vi "valve_command.vi"(8 "Error IN":errorcluster, 9 "Command option":string, 10 "COMMANDS":T1(ring), 11 "VALVE PORT IN":refnum<visa-resource-name>="COM1") -> (0 "Error OUT":errorcluster, 2 "read buffer":string, 3 "VALVE PORT OUT":refnum<visa-resource-name>)   [LabVIEW 2013]
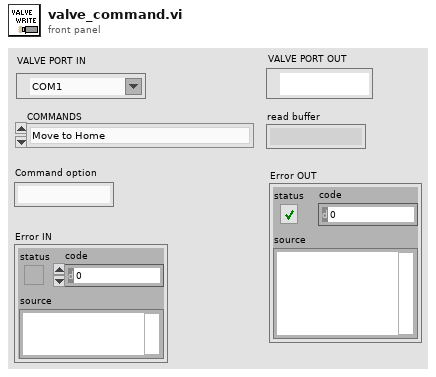
[diagram p1: front panel]
types:
  T1 = enum16{"Move to Home", "Set Positions", "Set Actuator Mode", "OTHER", "Set Direction", "CW Move", "CCW Move"}
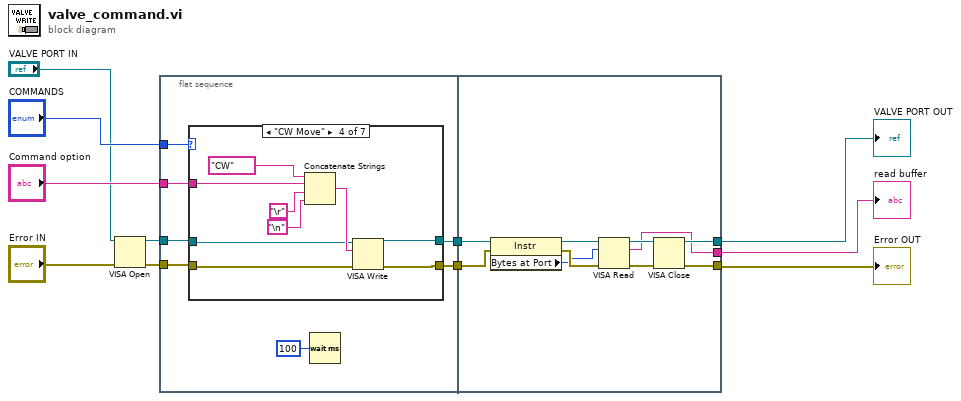
[diagram p0: block diagram]
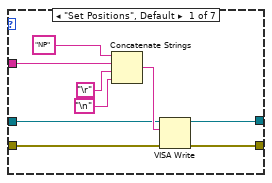
[diagram p2: hidden frame]
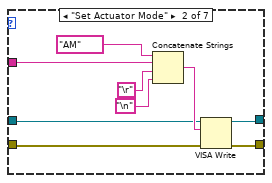
[diagram p3: hidden frame]
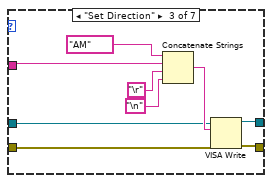
[diagram p4: hidden frame]
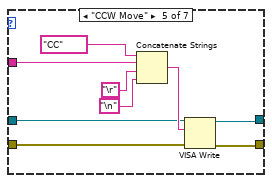
[diagram p5: hidden frame]
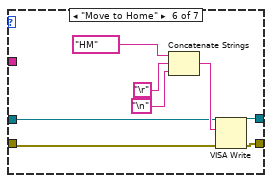
[diagram p6: hidden frame]
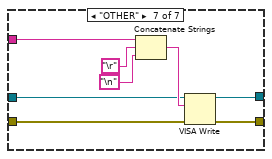
[diagram p7: hidden frame]
diagram:
  n1 = VISA Open(error in (no error)="Error IN", VISA resource name="VALVE PORT IN") -> (VISA resource name=w6:refnum<visa-resource-name>, error out=w4:errorcluster)  [unwired: 3 in]
  n2 = flat-sequence {
    tunnel: "COMMANDS" -> [w18]
    tunnel: "Command option" -> [w17]
    tunnel: w6 -> [w14]
    tunnel: w4 -> [w13]
    tunnel: [w16] -> w3
    tunnel: [w15] -> w2
    tunnel: [w81] -> w8
    tunnel: [w82] -> w9
    tunnel: w3 -> [w83]
    tunnel: w2 -> [w84]
    tunnel: [w80] -> w1
    frame #0 {
      n3 = case shown="\"CW Move\"" w18 {
        tunnel: w14 -> [w21 w29 w41 w49 w59 w69 w75]
        tunnel: w13 -> [w23 w32 w40 w48 w58 w66 w74]
        tunnel: w17 -> [w19 w28 w37 w50 w55 _ w78]
        tunnel: [w20 w30 w38 w46 w57 w68 w73] -> w15
        tunnel: [w22 w31 w39 w47 w56 w67 w72] -> w16
        frame "Set Positions", Default {
          n4 = Concatenate Strings("NP" ("write buffer 2"), w19, "\r", "\n") -> (w27:string)
          n5 = VISA Write(VISA resource name=w21, write buffer=w27, error in (no error)=w23) -> (VISA resource name out=w20:refnum<visa-resource-name>, error out=w22:errorcluster)  [unwired: 1 out]
        }
        frame "Set Actuator Mode" {
          n6 = Concatenate Strings("AM" ("write buffer 2"), w28, "\r", "\n") -> (w33:string)
          n7 = VISA Write(VISA resource name=w29, write buffer=w33, error in (no error)=w32) -> (VISA resource name out=w30:refnum<visa-resource-name>, error out=w31:errorcluster)  [unwired: 1 out]
        }
        frame "Set Direction" {
          n8 = Concatenate Strings("AM" ("write buffer 2"), w37, "\r", "\n") -> (w42:string)
          n9 = VISA Write(VISA resource name=w41, write buffer=w42, error in (no error)=w40) -> (VISA resource name out=w38:refnum<visa-resource-name>, error out=w39:errorcluster)  [unwired: 1 out]
        }
        frame "CW Move" {
          n10 = Concatenate Strings("CW" ("write buffer 2"), w50, "\r", "\n") -> (w51:string)
          n11 = VISA Write(VISA resource name=w49, write buffer=w51, error in (no error)=w48) -> (VISA resource name out=w46:refnum<visa-resource-name>, error out=w47:errorcluster)  [unwired: 1 out]
        }
        frame "CCW Move" {
          n12 = Concatenate Strings("CC" ("write buffer 2"), w55, "\r", "\n") -> (w60:string)
          n13 = VISA Write(VISA resource name=w59, write buffer=w60, error in (no error)=w58) -> (VISA resource name out=w57:refnum<visa-resource-name>, error out=w56:errorcluster)  [unwired: 1 out]
        }
        frame "Move to Home" {
          n14 = Concatenate Strings("HM" ("write buffer 2"), "\r", "\n") -> (w71:string)
          n15 = VISA Write(VISA resource name=w69, write buffer=w71, error in (no error)=w66) -> (VISA resource name out=w68:refnum<visa-resource-name>, error out=w67:errorcluster)  [unwired: 1 out]
        }
        frame "OTHER" {
          n16 = Concatenate Strings(w78, "\r", "\n") -> (w79:string)
          n17 = VISA Write(VISA resource name=w75, write buffer=w79, error in (no error)=w74) -> (VISA resource name out=w73:refnum<visa-resource-name>, error out=w72:errorcluster)  [unwired: 1 out]
        }
      }
      n18 = Wait (ms)(milliseconds to wait=u32 100) -> ()  [unwired: 1 out]
    }
    frame #1 {
      n19 = property class="Instr"(reference=w84, error in=w83) -> (reference out=w86:refnum<visa-resource-name>, error out=w87:errorcluster, "Bytes at Port"=w85:u32)
      n20 = VISA Read(VISA resource name=w86, byte count=w85, error in (no error)=w87) -> (VISA resource name out=w81:refnum<visa-resource-name>, read buffer=w80:string, error out=w88:errorcluster)  [unwired: 1 out]
      n21 = VISA Close(VISA resource name=w81, error in (no error)=w88) -> (error out=w82:errorcluster)
    }
  }
  "VALVE PORT OUT" <- w8
  "Error OUT" <- w9
  "read buffer" <- w1
